vi "SkalaToPic.vi"(4 "error in (no error)":errorcluster, 5 "nazwa pliku zdjęcia":string, 6 "rainbow array":u32[](array[numeric]), 7 "Katalog z plikami":path) -> (0 "error out":errorcluster, 1 "Bottom prost.":i32, 2 "rozdzielczość obrazu pomniejszona o 30px":i32, 3 "Image Out":T1(plugin-control))   [LabVIEW 2009]
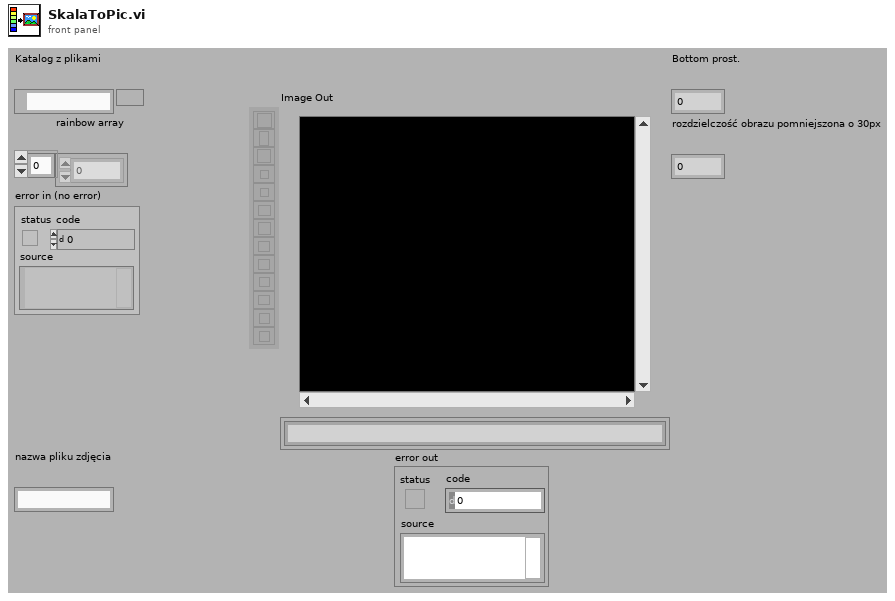
[diagram p1: front panel]
types:
  T1 = typedef "IMAQ Image.ctl" = refnum<image>
  T2 = cluster{"Left":i32, "Top":i32, "Right":i32, "Bottom":i32}
  T3 = typedef "Image Type" = u32
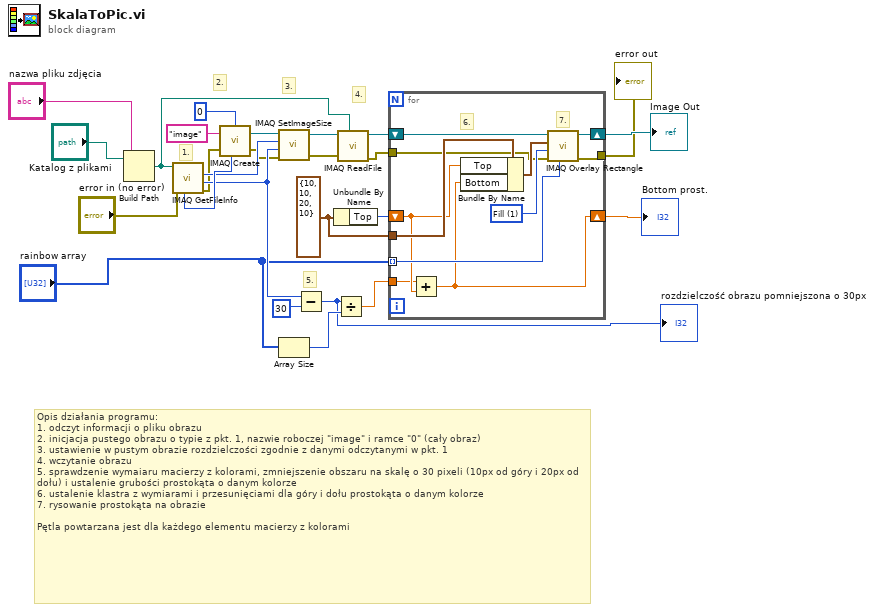
[diagram p0: block diagram]
diagram:
  w16 = T2 {"Left"=10, "Top"=10, "Right"=20, "Bottom"=10} ("Rectangle")
  # "Opis działania programu:\n1. odczyt informacji o pliku obrazu\n2. inicjacja pustego obrazu o typie z pkt. 1, nazwie roboczej \"image\" i ramce \"0\" (cały obraz)\n3. ustawienie w pustym obrazie rozdzielczości zgodnie z danymi odczytanymi w pkt. 1\n4. wczytanie obrazu\n5. sprawdzenie wymaiaru macierzy z kolorami, zmniejszenie obszaru na skalę o 30 pixeli (10px od góry i 20px od dołu) i ustalenie grubości prostokąta o danym kolorze\n6. ustalenie klastra z wymiarami i przesunięciami dla góry i dołu prostokąta o danym kolorze\n7. rysowanie prostokąta na obrazie\n\nPętla powtarzana jest dla każdego elementu macierzy z kolorami"
  # "5."
  # "4."
  # "3."
  # "2."
  # "1."
  n1 = Build Path(base path="Katalog z plikami", name or relative path="nazwa pliku zdjęcia") -> (appended path=w26:path)
  n2 = call "IMAQ GetFileInfo"("error in (no error)"="error in (no error)", "File Path"=w26) -> ("error out"=w6:errorcluster, "Y Resolution"=w14:i32, "X Resolution"=w20:i32, "Image Type"=w23:T3)  [unwired: 3 in, 3 out]
  n3 = call "IMAQ Create"("Border Size"=0, "Image Name"="image", "Image Type"=w23, "error in (no error)"=w6) -> ("New Image"=w22:T1, "error out"=w5:errorcluster)  [unwired: 1 in]
  n4 = call "IMAQ SetImageSize"("error in (no error)"=w5, "Y Resolution"=w14, "X Resolution"=w20, "Image"=w22) -> ("error out"=w4:errorcluster, "Image Out"=w21:T1)  [unwired: 1 in]
  n5 = Array Size(array="rainbow array") -> (size(s)=w15:i32)
  n6 = Subtract(x=w14, y=30) -> (x-y=w12:i32)
  "rozdzielczość obrazu pomniejszona o 30px" <- w12
  n7 = Unbundle By Name(w16) -> ("Top"=w17:i32)
  n8 = Divide(x=w12, y=w15) -> (x/y=w13:dbl)
  n9 = call "IMAQ ReadFile"("File Path"=w26, "error in (no error)"=w4, "Image"=w21) -> ("error out"=w3:errorcluster, "Image Out"=w19:T1)  [unwired: 4 in, 3 out]
  n10 = for {
    shift-right: [w35] -> w18
    shift-left: w19 -> [w36]
    tunnel: "rainbow array" -> [w34] mode=indexing
    shift-right: [w30] -> w10
    shift-left: w17 -> [w32]
    tunnel: w16 -> [w33]
    tunnel: w13 -> [w29]
    tunnel: w3 -> [w28]
    tunnel: [w27] -> w2
    w37 = u32 1 items=["Frame", "Fill", "Highlight"] ("Drawing Mode (Frame)")
    # "7."
    # "6."
    n11 = Add(x=w29, y=w32) -> (x+y=w30:dbl)
    n12 = Bundle By Name(cluster=w33, "Top"=w32, "Bottom"=w30) -> (w31:T2)
    n13 = call "IMAQ Overlay Rectangle"("Color"=w34, "error in (no error)"=w28, "Drawing Mode (Frame)"=w37, "Rectangle"=w31, "Image"=w36) -> ("error out"=w27:errorcluster, "Image Out"=w35:T1)  [unwired: 5 in]
  }
  "Image Out" <- w18
  "Bottom prost." <- w10
  "error out" <- w2
